vi "Write Student Info.vi"(8 "Error In":errorcluster, 10 "Student Info":T1, 11 "Path In":path) -> (0 "Error Out":errorcluster, 3 "Path Out":path)   [LabVIEW 2014]
uses:
  Ctls/Student Info.ctl
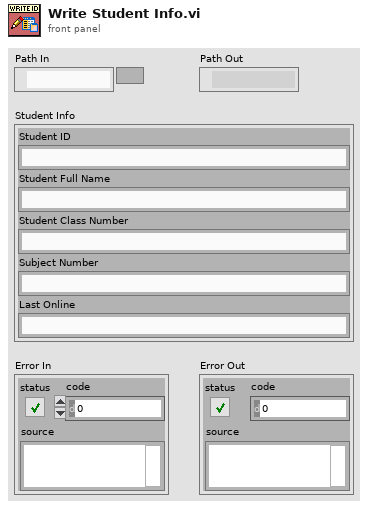
[diagram p1: front panel]
types:
  T1 = typedef "Student Info.ctl" = cluster{"Student ID":string, "Student Full Name":string, "Student Class Number":string, "Subject Number":string, "Last Online":string}
  T2 = enum16{"open", "replace", "create", "open or create", "replace or create", "replace or create with confirmation"}
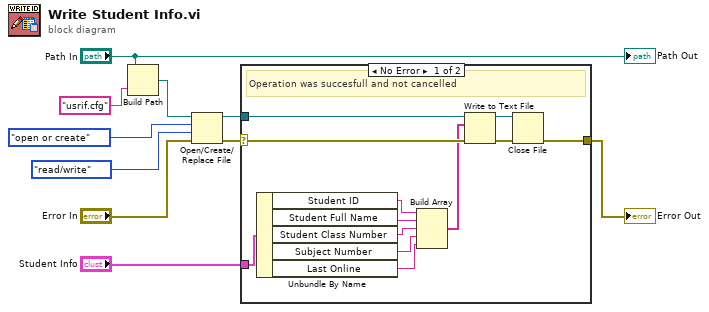
[diagram p0: block diagram]
diagram:
  n1 = Build Path(base path="Path In", name or relative path="usrif.cfg") -> (appended path=w2:path)
  n2 = Open/Create/Replace File(file path (use dialog)=w2, error in="Error In", operation (0:open)=T2."open or create", access (0:read/write)=enum16{"read/write", "read-only", "write-only"}."read/write") -> (refnum out=w8:refnum<file>, error out=w7:errorcluster)  [unwired: 2 in, 1 out]
  n3 = case shown="No Error" w7 {
    selector: w7 -> [w21 w23]
    tunnel: w8 -> [w22 _]
    tunnel: [w18 w23] -> w9
    tunnel: "Student Info" -> [w17 _]
    frame No Error {
      # "Operation was succesfull and not cancelled"
      n4 = Unbundle By Name(w17) -> ("Student ID"=w16:string, "Student Full Name"=w15:string, "Student Class Number"=w14:string, "Subject Number"=w13:string, "Last Online"=w12:string)
      n5 = Build Array(w16, w15, w14, w13, w12) -> (w11:string[])
      n6 = Write to Text File(file (use dialog)=w22, text=w11, error in=w21) -> (refnum out=w20:refnum<file>, error out=w19:errorcluster)  [unwired: 1 in, 1 out]
      n7 = Close File(refnum=w20, error in=w19) -> (error out=w18:errorcluster)  [unwired: 1 out]
    }
    frame Error {
      # "Error to find file. Default to create new file"
    }
  }
  "Error Out" <- w9
  "Path Out" <- "Path In"
